vi "Actor Core.vi"(8 "error in":errorcluster, 11 "LabGUI in":refnum<class "LabGUI.lvclass">) -> (0 "error out":errorcluster, 3 "Actor out":refnum<class "Actor.lvclass">)   [LabVIEW 2019, in "LabGUI.lvlib" / "LabGUI.lvclass"]
doc: "(<B>Filename</B>: Actor Framework.lvlib:Actor.lvclass:Actor Core.vi)\n\nReceives messages to the actor, reacts to them, and initiates any error handling that may shut the actor down.\n\nDescendant classes may override this VI to append parallel tasks for the actor to complete while it handles messages. Overrides use the Call Parent Method node."
uses:
  LabGUI.lvclass
  C:/Program Files (x86)/National Instruments/LabVIEW 2019/vi.lib/MGI/Panel Manager/Panel Actor/Panel Actor/Panel Actor.lvclass
  <vilib>/ActorFramework/Actor/Actor.lvclass
  LabGUI.lvclass/LabGUI.ctl
  MiniGUI/MiniGUI/MiniGUI.lvclass
  LabGUI Messages/Map MiniGUIs Msg/Map MiniGUIs Msg.lvclass/Map MiniGUIs Msg.ctl
  <vilib>/ActorFramework/Message Enqueuer/Message Enqueuer.lvclass/Message Enqueuer.ctl
  LabGUI Messages/Show MiniGUI Msg/Show MiniGUI Msg.lvclass/Show MiniGUI Msg.ctl
  <vilib>/ActorFramework/Message Enqueuer/Enqueue.vi
  <vilib>/MGI/Panel Manager/Panel/Panel/Subpanel/Subpanel.lvclass
  C:/Program Files (x86)/National Instruments/LabVIEW 2019/vi.lib/MGI/Panel Manager/Panel/Panel/Panel.lvclass
  LabGUI Messages/Map MiniGUIs Msg/Map MiniGUIs Msg.lvclass
  C:/Program Files (x86)/National Instruments/LabVIEW 2019/vi.lib/ActorFramework/Message/Message.lvclass
  LabGUI Messages/Show MiniGUI Msg/Show MiniGUI Msg.lvclass
  <vilib>/ActorFramework/Stop Msg/Stop Msg.lvclass
  <vilib>/MGI/Panel Manager/Panel/Panel/Subpanel/Subpanel.vi
  <vilib>/ActorFramework/Message Priority Queue/Priority Enqueue.vi
  <vilib>/MGI/Panel Manager/Panel Actor/Panel Actor/Panel Actor.lvclass
  <vilib>/MGI/Panel Manager/Panel/Panel.lvlib
  <vilib>/nisyscfg/nisyscfg.lvlib
panel:
  out "Title":string
  in  "Refresh":bool
  in  "Detected Systems":i32(listbox)
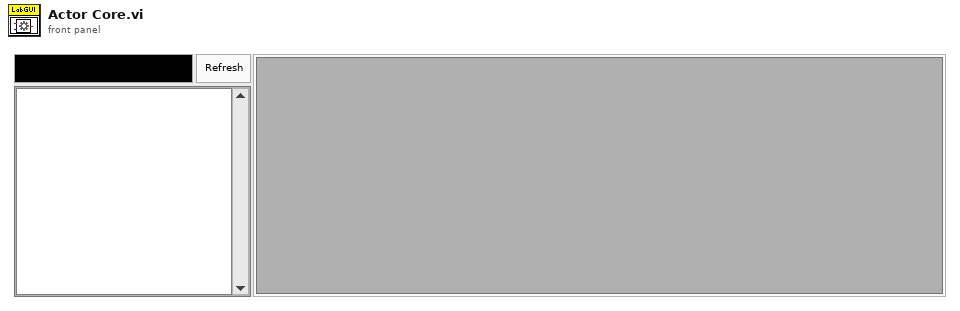
[diagram p1: front panel]
types:
  T1 = enum32{"Invalid", "Standard", "Closed", "Hidden", "Minimized", "Maximized"}
  T2 = typedef "Panel.lvlib/Panel Helper.lvclass/Events.ctl" = enum16{"Initialized", "Shown", "Hidden", "Closed"}
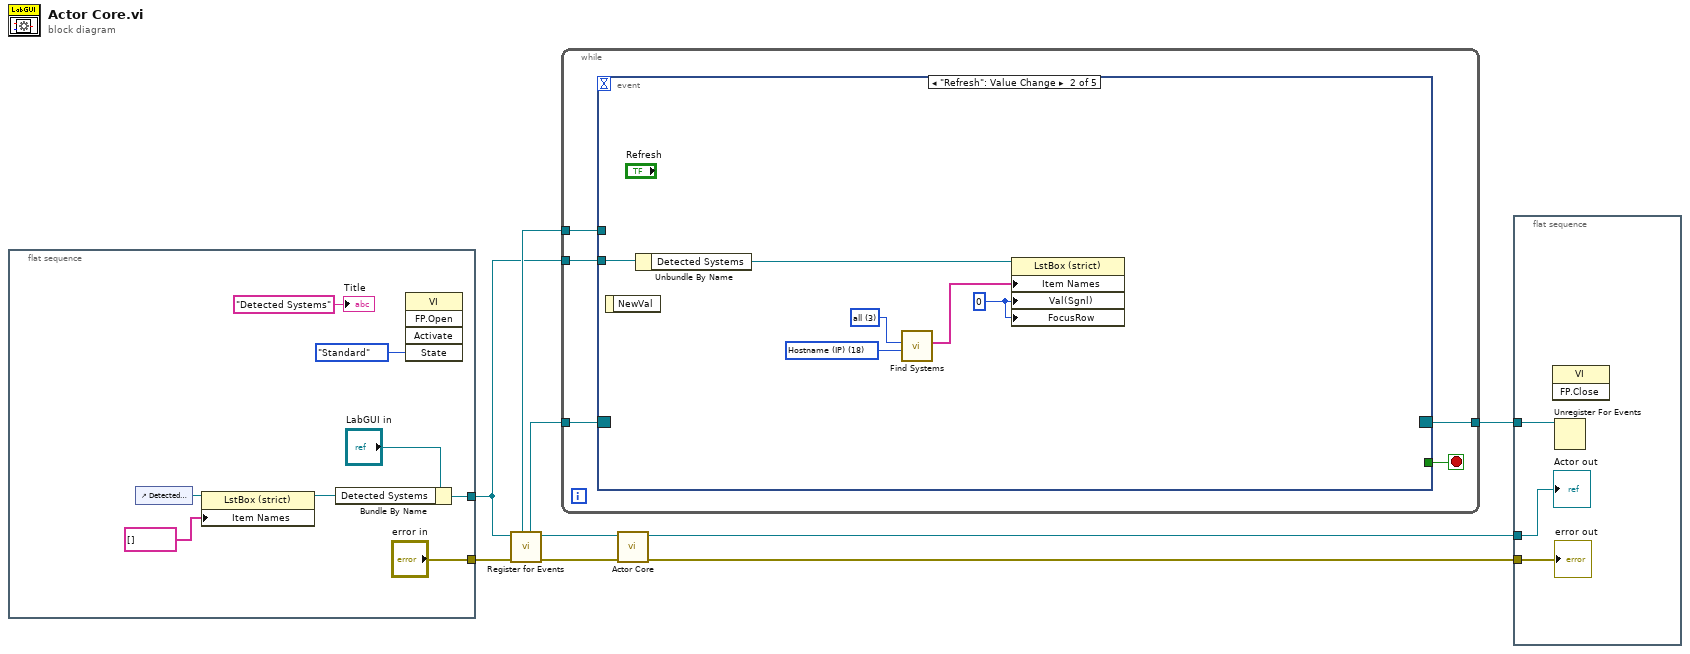
[diagram p0: block diagram]
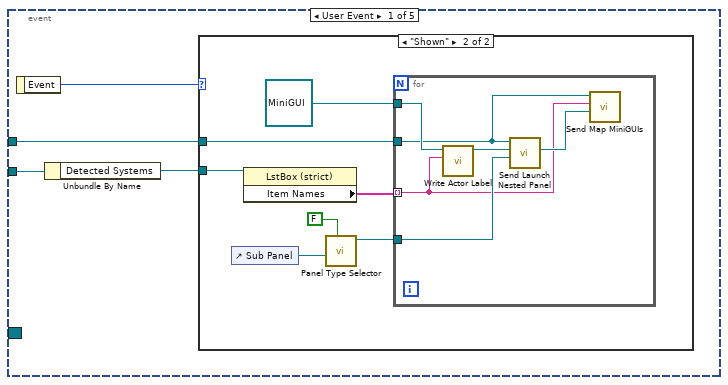
[diagram p2: hidden frame]
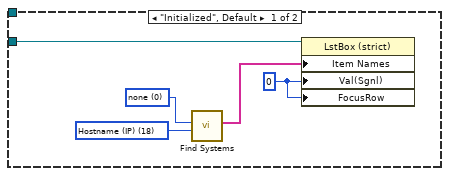
[diagram p3: hidden frame]
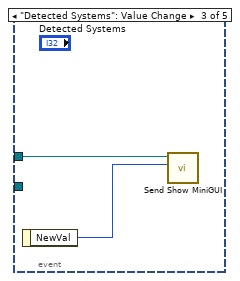
[diagram p4: hidden frame]
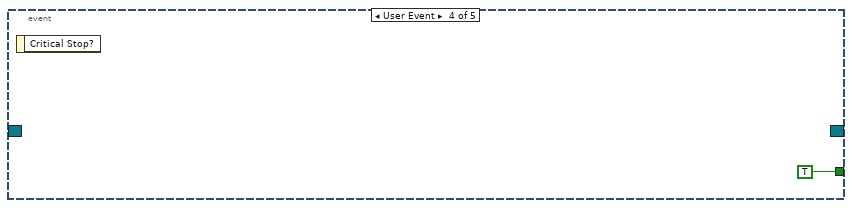
[diagram p5: hidden frame]
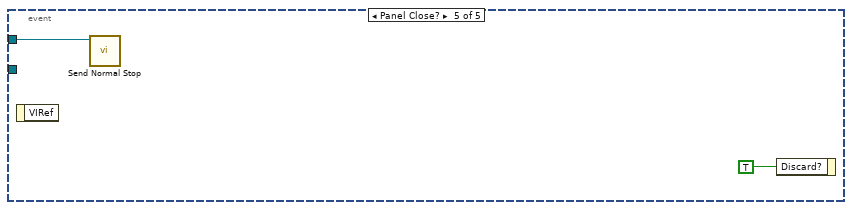
[diagram p6: hidden frame]
diagram:
  n1 = flat-sequence {
    tunnel: ["error in"] -> w2
    tunnel: [w13] -> w1
    frame #0 {
      n2 = control-ref of="Detected Systems"() -> (w12:refnum<vi>)
      n3 = property class="LstBox (strict)"(reference=w12, "Item Names"=string[] []) -> (reference out=w10:refnum<vi>)  [unwired: 1 in, 1 out]
      n4 = Bundle By Name(cluster="LabGUI in", "Detected Systems"=w10) -> (w13:refnum<class "LabGUI.lvclass">)
      n5 = invoke class="VI" method="FP.Open"("State"=T1."Standard") -> ()  [unwired: 4 in, 5 out]
      "Title" <- "Detected Systems" ("Title")
    }
  }
  n6 = call <vilib>:"Register for Events.vi"("Error In"=w2, "Panel Actor in"=w1) -> ("Error Out"=w7:errorcluster, "Panel Actor out"=w6:refnum<class "LabGUI.lvclass">, "Pnl Actor"=w5:refnum<event-registration>, "Self Enqueuer"=w4:refnum<class "Message Enqueuer.lvclass">)  [unwired: 6 in]
  n7 = while {
    tunnel: w5 -> [w22]
    tunnel: w4 -> [w21]
    tunnel: [w19] -> w3
    tunnel: w1 -> [w18]
    stop <- w20 stop-if-true
    n8 = event shown="[1] \"Refresh\": Value Change" {
      selector: w22 -> [_ _ _ _ _]
      dyn-events: [_ _ _ _ _] -> w19
      timeout: _ -> [_ _ _ _ _]
      tunnel: w21 -> [w25 _ w51 _ w54]
      tunnel: [_ _ _ TRUE _] -> w20
      tunnel: w18 -> [w24 w46 _ _ _]
      event User Event {
        n9 = event-data() -> ("Event"=w26:T2)  [unwired: 1 in]
        n10 = Unbundle By Name(w24) -> ("Detected Systems"=w23:refnum<vi>)
        n11 = case shown="\"Shown\"" w26 {
          tunnel: w25 -> [_ w34]
          tunnel: w23 -> [w29 w33]
          frame "Initialized", Default {
            w28 = 0 ("Value (Signaling)")
            w30 = u32 0 items=["none"=0, "only if online"=1, "all"=3] ("Include Cached Results (all)")
            w31 = u32 18 items=["Hostname"=16, "Hostname (IP)"=18, "Hostname (MAC)"=19, "IP"=32, "IP (Hostname)"=33, "IP (MAC)"=35, "MAC"=48, "MAC (Hostname)"=49, "MAC (IP)"=50] ("Output (Hostname and IP)")
            n12 = call <vilib>:"Find Systems.vi"("Output (Hostname and IP)"=w31, "Include Cached Results (all)"=w30) -> ("Detected Systems"=w27:string[])  [unwired: 7 in, 2 out]
            n13 = property class="LstBox (strict)"(reference=w29, "Item Names"=w27, "Val(Sgnl)"=w28, "FocusRow"=w28) -> ()  [unwired: 1 in, 2 out]
          }
          frame "Shown" {
            n14 = control-ref of="Sub Panel"() -> (w38:refnum<vi>)
            n15 = property class="LstBox (strict)"(reference=w33) -> ("Item Names"=w32:string[])  [unwired: 1 in, 2 out]
            n16 = call-poly <vilib>:"Panel Type Selector.vi"("Autoshow? (T)"=FALSE, "Sub Panel"=w38) -> ("Subpanel Out"=w36:refnum<class "Subpanel.lvclass">)  [unwired: 8 in, 1 out]
            n17 = for {
              tunnel: w32 -> [w39] mode=indexing
              tunnel: w36 -> [w43]
              tunnel: w34 -> [w41]
              tunnel: refnum<class "MiniGUI.lvclass"> refnum ("MiniGUI.lvlib:MiniGUI.lvclass") -> [w42]
              n18 = call-dynamic "Write Actor Label.vi"("Actor Label"=w39, "Monitored Actor in"=w42) -> ("Monitored Actor out"=w44:refnum<class "MiniGUI.lvclass">)  [unwired: 8 in, 1 out]
              n19 = call <vilib>:"Send Launch Nested Panel.vi"("Panel"=w43, "Nested Panel Actor"=w44, "Self Enqueuer in"=w41) -> ("Nested Actor's Enqueuer"=w40:refnum<class "Message Enqueuer.lvclass">)  [unwired: 7 in, 1 out]
              n20 = call "Send Map MiniGUIs.vi"("MiniGUI"=w40, "key"=w39, "Message Enqueuer"=w41) -> ()  [unwired: 7 in, 2 out]
            }
          }
        }
      }
      event "Refresh": Value Change {
        w49 = 0 ("Value (Signaling)")
        w47 = u32 3 items=["none"=0, "only if online"=1, "all"=3] ("Include Cached Results (all)")
        w48 = u32 18 items=["Hostname"=16, "Hostname (IP)"=18, "Hostname (MAC)"=19, "IP"=32, "IP (Hostname)"=33, "IP (MAC)"=35, "MAC"=48, "MAC (Hostname)"=49, "MAC (IP)"=50] ("Output (Hostname and IP)")
        n21 = event-data() -> ()  [unwired: 1 in, 1 out]
        n22 = Unbundle By Name(w46) -> ("Detected Systems"=w45:refnum<vi>)
        n23 = call <vilib>:"Find Systems.vi"("Output (Hostname and IP)"=w48, "Include Cached Results (all)"=w47) -> ("Detected Systems"=w50:string[])  [unwired: 7 in, 2 out]
        n24 = property class="LstBox (strict)"(reference=w45, "Item Names"=w50, "Val(Sgnl)"=w49, "FocusRow"=w49) -> ()  [unwired: 1 in, 2 out]
      }
      event "Detected Systems": Value Change {
        n25 = event-data() -> ("NewVal"=w52:i32)  [unwired: 1 in]
        n26 = call "Send Show MiniGUI.vi"("MiniGUI Index"=w52, "Message Enqueuer"=w51) -> ()  [unwired: 8 in, 2 out]
      }
      event User Event {
        n27 = event-data() -> ()  [unwired: 1 in, 1 out]
      }
      event Panel Close? {
        n28 = event-data() -> ()  [unwired: 1 in, 1 out]
        n29 = call <vilib>:"Send Normal Stop.vi"("Message Enqueuer"=w54) -> ()  [unwired: 10 in, 1 out]
        n30 = event-data("Discard?"=TRUE) -> ()  [unwired: 1 in, 1 out]
      }
    }
  }
  n31 = call-parent "Actor Core.vi"("error in"=w7, "Panel Actor in"=w6) -> ("error out"=w9:errorcluster, "Actor out"=w8:refnum<class "Actor.lvclass">)  [unwired: 8 in]
  n32 = flat-sequence {
    tunnel: w9 -> [w58]
    tunnel: w8 -> [w57]
    tunnel: w3 -> [w56]
    frame #0 {
      n33 = invoke class="VI" method="FP.Close"() -> ()  [unwired: 3 in, 3 out]
      n34 = Unregister For Events(event registration refnum=w56) -> ()  [unwired: 1 in, 1 out]
      "error out" <- w58
      "Actor out" <- w57
    }
  }
